vi "toXml.vi"(8 "error in (no error)":errorcluster, 11 "DataPointScript in":refnum<class "DataPointScript.lvclass">) -> (0 "error out":errorcluster, 2 "dataPointXml":refnum<class "xmlNode.lvclass">, 3 "DataPointScript out":refnum<class "DataPointScript.lvclass">)   [LabVIEW 2009, in "Tools.lvlib" / "Scripting.lvlib" / "DataPointScript.lvclass"]
uses:
  DataPointScript.lvclass
  xmlNode/xmlNode.lvclass
  DataPointScript.lvclass/DataPointScript.ctl
  ScriptingEvent/ScriptEventList/ScriptEventList.lvclass
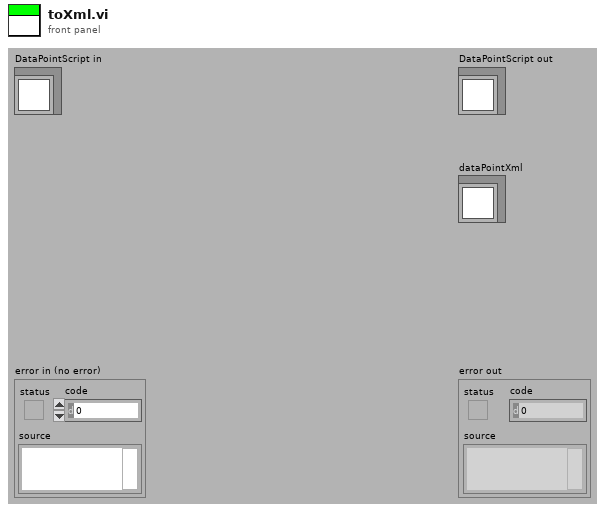
[diagram p1: front panel]
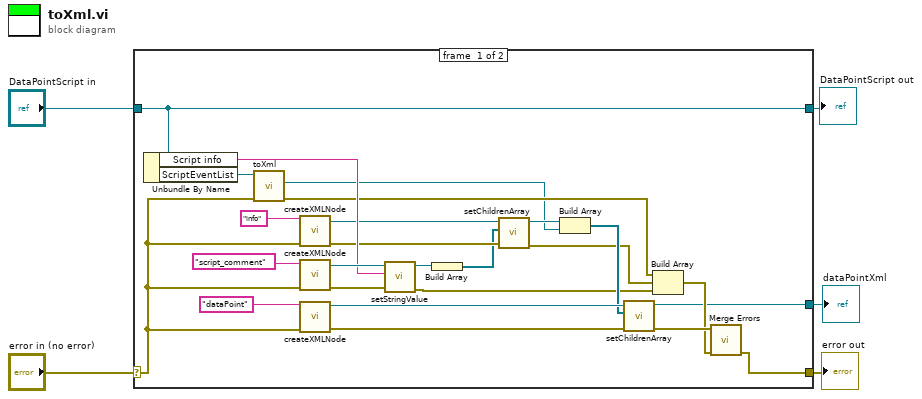
[diagram p0: block diagram]
diagram:
  n1 = case shown="No Error" "error in (no error)" {
    selector: "error in (no error)" -> [w18 w32]
    tunnel: [w8 w32] -> w4
    tunnel: [w30 w31] -> w2
    tunnel: "DataPointScript in" -> [w30 w31]
    tunnel: [w7 _] -> w1
    frame #0 {
      n2 = Unbundle By Name(w30) -> ("Script info"=w24:string, "ScriptEventList"=w28:refnum<class "ScriptEventList.lvclass">)
      n3 = call "toXml.vi"("error in (no error)"=w18, "ScriptEventList in"=w28) -> ("error out"=w10:errorcluster, "event_listXml"=w6:refnum<class "xmlNode.lvclass">)  [unwired: 7 in, 1 out]
      n4 = call "createXMLNode.vi"("error in (no error)"=w18, "name"="info") -> ("error out"=w21:errorcluster, "xmlNode out"=w22:refnum<class "xmlNode.lvclass">)  [unwired: 8 in]
      n5 = call "createXMLNode.vi"("error in (no error)"=w18, "name"="script_comment") -> ("error out"=w25:errorcluster, "xmlNode out"=w26:refnum<class "xmlNode.lvclass">)  [unwired: 8 in]
      n6 = call "createXMLNode.vi"("error in (no error)"=w18, "name"="dataPoint") -> ("error out"=w14:errorcluster, "xmlNode out"=w17:refnum<class "xmlNode.lvclass">)  [unwired: 8 in]
      n7 = call-dynamic "setStringValue.vi"("error in (no error)"=w25, "stringValue"=w24, "xmlNode.lvclass in"=w26) -> ("error out"=w12:errorcluster, "xmlNode.lvclass out"=w23:refnum<class "xmlNode.lvclass">)  [unwired: 7 in]
      n8 = Build Array(w23) -> (w20:refnum<class "xmlNode.lvclass">[])
      n9 = call-dynamic "setChildrenArray.vi"("error in (no error)"=w21, "Children"=w20, "xmlNode.lvclass in"=w22) -> ("error out"=w11:errorcluster, "xmlNode.lvclass out"=w16:refnum<class "xmlNode.lvclass">)  [unwired: 7 in]
      n10 = Build Array(w16, w6) -> (w15:refnum<class "xmlNode.lvclass">[])
      n11 = call-dynamic "setChildrenArray.vi"("error in (no error)"=w14, "Children"=w15, "xmlNode.lvclass in"=w17) -> ("error out"=w13:errorcluster, "xmlNode.lvclass out"=w7:refnum<class "xmlNode.lvclass">)  [unwired: 7 in]
      n12 = Build Array(w10, w11, w12) -> (w9:errorcluster[])
      n13 = call <vilib>:"Merge Errors.vi"("error array in"=w9, "error in 1 (no error)"=w13) -> ("error out"=w8:errorcluster)  [unwired: 5 in]
    }
    frame #1 {
    }
  }
  "error out" <- w4
  "DataPointScript out" <- w2
  "dataPointXml" <- w1
